vi "valves_oil_suction.vi"(0 "PID Gains Cluster Ref":refnum<vi>, 1 "Accept Autotune":bool, 2 "Controller Toggle (Manual Mode)":bool, 3 "Valve Manual Adjust":dbl, 5 "Slide Refnum in":refnum<vi>, 7 "file (use dialog)":path, 9 "Desired Setpoint":dbl, 11 "PID gains":T2, 12 "Current Process Variable Value":dbl, 13 "autotune? (F)":bool, 14 "Reinitialize Controller":bool) -> (4 "output to valve":dbl, 6 "output to slide":dbl, 8 "tuning completed?":bool, 10 "plant parameters out":T1, 15 "PID gains out":T2)   [LabVIEW 2017]
uses:
  <vilib>/addons/control/pid/autopid.llb/PID autotuning parameters (FO).ctl
  <vilib>/addons/control/pid/NI_PID_autopid.lvlib
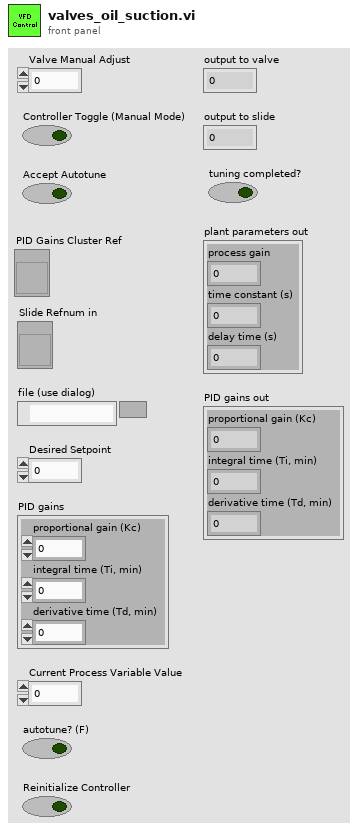
[diagram p1: front panel]
types:
  T1 = cluster{"process gain":dbl, "time constant (s)":dbl, "delay time (s)":dbl}
  T2 = cluster{"proportional gain (Kc)":dbl, "integral time (Ti, min)":dbl, "derivative time (Td, min)":dbl}
  T3 = typedef "NI_PID_autopid.lvlib/PID autotuning parameters (FO).ctl" = cluster{"type of controller":u16, "time constant factor":dbl, "step amplitude":dbl}
  T4 = enum8{"Enabled", "Disabled", "Disabled and Grayed Out"}
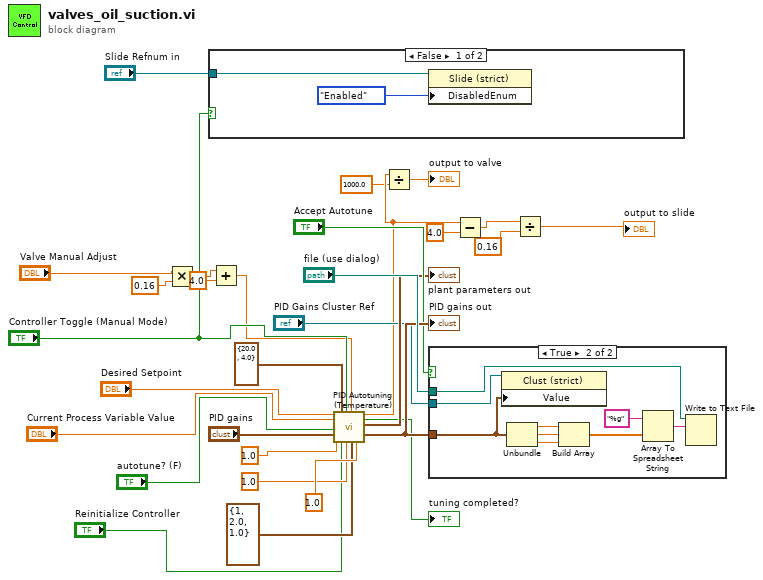
[diagram p0: block diagram]
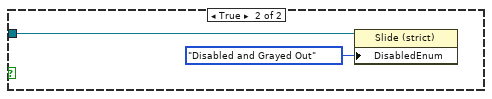
[diagram p3: hidden frame]
diagram:
  n1 = Multiply(x="Valve Manual Adjust", y=0.16) -> (x*y=w10:dbl)
  n2 = case shown="False" "Controller Toggle (Manual Mode)" {
    tunnel: "Slide Refnum in" -> [w31 w34]
    frame False {
      n3 = property on="Property Node" class="Slide (strict)"(reference=w31, "DisabledEnum"=T4."Enabled" ("Disabled")) -> ()  [unwired: 1 in, 2 out]
    }
    frame True {
      n4 = property on="Property Node" class="Slide (strict)"(reference=w34, "DisabledEnum"=T4."Disabled and Grayed Out" ("Disabled")) -> ()  [unwired: 1 in, 2 out]
    }
  }
  n5 = Add(x=w10, y=4.0) -> (x+y=w8:dbl)
  n6 = call <vilib>:"PID Autotuning (Temperature).vi"("desired temperature"="Desired Setpoint", "measured temperature"="Current Process Variable Value", "autotune? (F)"="autotune? (F)", "PID gains in"="PID gains", "dt (s)"=1.0, "output range"=cluster{"output high":dbl, "output low":dbl} {"output high"=20.0, "output low"=4.0}, "reinitialize? (F)"="Reinitialize Controller", "auto? (T)"="Controller Toggle (Manual Mode)", "beta"=1.0, "manual control"=w8, "autotuning parameters"=T3 {"type of controller"=1, "time constant factor"=2.0, "step amplitude"=1.0}, "alpha"=1.0) -> ("output"=w2:dbl, "tuning completed?"=→"tuning completed?":bool, "plant parameters out"=→"plant parameters out":T1, "PID gains out"=w28:T2)  [unwired: 4 in]
  "PID gains out" <- w28
  n7 = Divide(x=w2, y=1000.0) -> (x/y=→"output to valve":dbl)
  n8 = case shown="True" "Accept Autotune" {
    tunnel: w28 -> [_ w43]
    tunnel: "file (use dialog)" -> [_ w36]
    tunnel: "PID Gains Cluster Ref" -> [_ w35]
    frame False {
    }
    frame True {
      n9 = property class="Clust (strict)"(reference=w35, "Value"=w43) -> ()  [unwired: 1 in, 2 out]
      n10 = Unbundle(w43) -> ("proportional gain (Kc)"=w42:dbl, "integral time (Ti, min)"=w41:dbl, "derivative time (Td, min)"=w40:dbl)
      n11 = Build Array(w42, w41, w40) -> (w39:dbl[])
      n12 = Array To Spreadsheet String(array=w39, 3:"%g" ("format string")) -> (spreadsheet string=w38:string)  [unwired: 1 in]
      n13 = Write to Text File(file (use dialog)=w36, text=w38) -> ()  [unwired: 2 in, 3 out]
    }
  }
  n14 = Subtract(x=w2, y=4.0) -> (x-y=w7:dbl)
  n15 = Divide(x=w7, y=0.16) -> (x/y=→"output to slide":dbl)
